vi "Wait For Device.vi"(0 "session in":refnum<class "Digitizer Control.lvclass">, 5 "error in (no error)":errorcluster, 7 "timeout (ms)":i32=5000) -> (14 "session out":refnum<class "Digitizer Control.lvclass">, 15 "io error":i32, 19 "error out":errorcluster)   [LabVIEW 2021, in "Digitizer Control.lvclass"]
doc: "Waits and blocks the data flow until the FlexRIO module I/O is ready.\n\nInputs:\n\n<B>session in</B>: The device session.\n\n<B>timeout</B>: The maximum amount of time, in milliseconds, this VI is allowed to wait for the FlexRIO module I/O to become ready.\n\nOutputs:\n\n<B>session out</B>: The device session passed on the <B>session in</B> input.\n\n<B>io error</B>: Error code indicating why the I/O module is not ready."
uses:
  Digitizer Control.lvclass
  Digitizer Control.lvclass/Digitizer Control.ctl
  <instrlib>/FlexRIO/API/Host/v1/NI FlexRIO API v1.lvlib
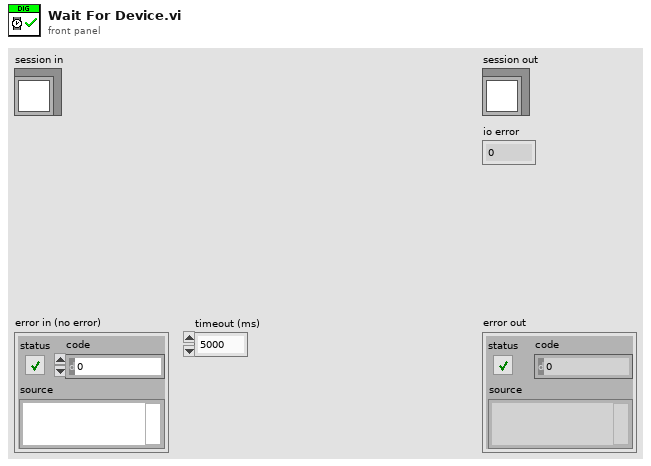
[diagram p1: front panel]
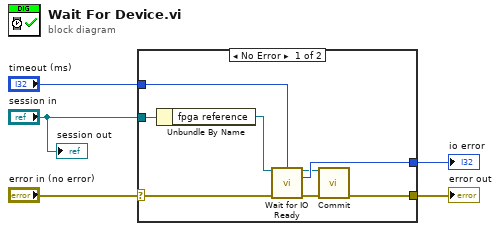
[diagram p0: block diagram]
diagram:
  n1 = case shown="No Error" "error in (no error)" {
    selector: "error in (no error)" -> [w12 w14]
    tunnel: "session in" -> [w13 _]
    tunnel: [w6 w14] -> w3
    tunnel: "timeout (ms)" -> [w10 _]
    tunnel: [w9 _] -> w1
    frame No Error {
      n2 = Unbundle By Name(w13) -> ("fpga reference"=w11:refnum<k20>)
      n3 = call <instrlib>:"Wait for IO Ready.vi"("fpga interface in"=w11, "timeout"=w10, "error in"=w12) -> ("fpga interface out"=w7:refnum<k20>, "io error"=w9:i32, "error out"=w8:errorcluster)  [unwired: 9 in, 1 out]
      n4 = call <instrlib>:"Commit.vi"("fpga interface in"=w7, "error in"=w8) -> ("error out"=w6:errorcluster)  [unwired: 12 in, 1 out]
    }
    frame Error {
    }
  }
  "error out" <- w3
  "io error" <- w1
  "session out" <- "session in"
